vi "InjectParent.vi"(8 "error in (no error)":errorcluster, 10 "Parent":refnum<vi>, 11 "CreateClass in":refnum<class "CreateClass.lvclass">) -> (0 "error out":errorcluster, 3 "CreateClass out":refnum<class "CreateClass.lvclass">)   [LabVIEW 2020, in "Mermaid.lvlib" / "CreateClass.lvclass"]
uses:
  CreateClass.lvclass
  CreateClass.lvclass/CreateClass.ctl
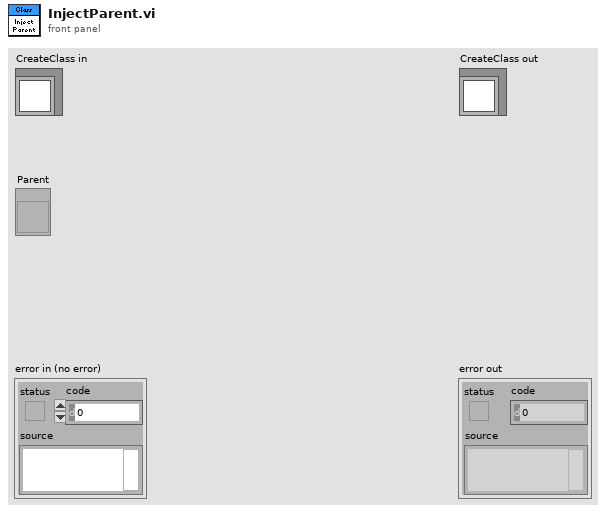
[diagram p1: front panel]
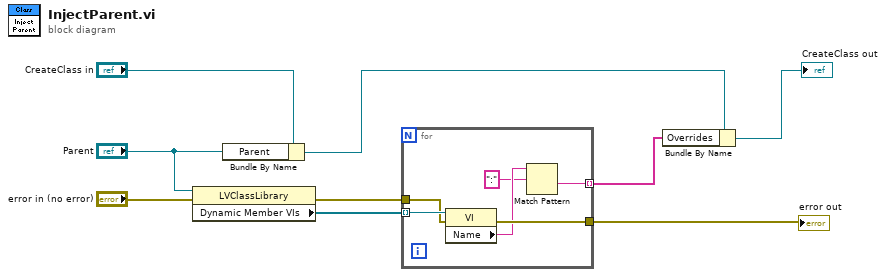
[diagram p0: block diagram]
diagram:
  n1 = property class="LVClassLibrary"(reference="Parent", error in="error in (no error)") -> (error out=w5:errorcluster, "Dynamic Member VIs"=w7:refnum<vi>[])  [unwired: 1 out]
  n2 = Bundle By Name(cluster="CreateClass in", "Parent"="Parent") -> (w2:refnum<class "CreateClass.lvclass">)
  n3 = for {
    tunnel: w7 -> [w15] mode=indexing
    tunnel: [w10] -> w3 mode=indexing
    tunnel: w5 -> [w14]
    tunnel: [w13] -> w4
    n4 = property class="VI"(reference=w15, error in=w14) -> (error out=w13:errorcluster, "Name"=w12:string)  [unwired: 1 out]
    n5 = Match Pattern(string=w12, regular expression=":") -> (after substring=w10:string)  [unwired: 1 in, 3 out]
  }
  "error out" <- w4
  n6 = Bundle By Name(cluster=w2, "Overrides"=w3) -> (→"CreateClass out":refnum<class "CreateClass.lvclass">)
